vi "AnalogInputVals.vi"(8 "error in (no error)":errorcluster, 11 "SerialPortRef":T1) -> (0 "error out":errorcluster, 2 "Array":bool[](array[boolean]), 3 "SerialRefOut":T1)   [LabVIEW 2015]
uses:
  <vilib>/Rock Robotics/WPI/SerialPort/WPI_SerialPortRef.ctl
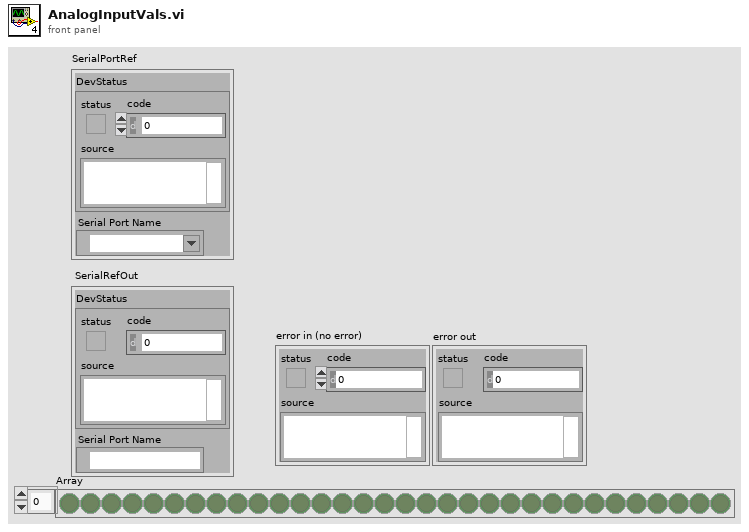
[diagram p1: front panel]
types:
  T1 = typedef "WPI_SerialPortRef.ctl" = cluster{"DevStatus":errorcluster, "Serial Port Name":refnum<visa-resource-name>}
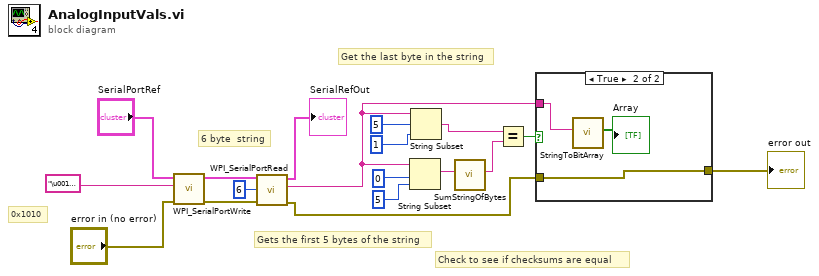
[diagram p0: block diagram]
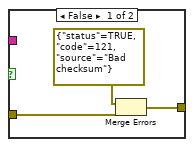
[diagram p2: hidden frame]
diagram:
  # "Check to see if checksums are equal"
  # "6 byte  string"
  # "Gets the first 5 bytes of the string"
  # "Get the last byte in the string"
  # "0x1010"
  n1 = call <vilib>:"WPI_SerialPortWrite.vi"("error in (no error)"="error in (no error)", "Buffer"="\u0010\u0010", "SerialPortRef"="SerialPortRef") -> ("error out"=w16:errorcluster, "SerialPortRef"=w13:T1)  [unwired: 6 in, 1 out]
  n2 = call <vilib>:"WPI_SerialPortRead.vi"("error in (no error)"=w16, "Num Bytes to Read"=u32 6, "SerialPortRef"=w13) -> ("error out"=w2:errorcluster, "Buffer"=w3:string, "SerialPortRef"=→"SerialRefOut":T1)  [unwired: 6 in]
  n3 = String Subset(string=w3, offset (0)=0, length (rest)=5 ("length (rest)")) -> (substring=w9:string)
  n4 = String Subset(string=w3, offset (0)=5, length (rest)=1 ("length (rest)")) -> (substring=w5:string)
  n5 = call "SumStringOfBytes.vi"("String Of Bytes"=w9) -> ("SumAsString"=w6:string)  [unwired: 10 in]
  n6 = Equal?(x=w5, y=w6) -> (x = y?=w4:bool)
  n7 = case shown="True" w4 {
    tunnel: w3 -> [_ w24]
    tunnel: [w21 w22] -> w1
    tunnel: w2 -> [w19 w22]
    frame False {
      n8 = Merge Errors(errorcluster {"status"=TRUE, "code"=121, "source"="Bad checksum"} ("error in"), w19) -> (w21:errorcluster)
    }
    frame True {
      n9 = call "StringToBitArray.vi"("string"=w24) -> ("Array"=→"Array":bool[])  [unwired: 10 in]
    }
  }
  "error out" <- w1
